vi "search_array_for_matches.vi"(9 "protocol selection ref":refnum<vi>, 10 "Protocol enum":T1, 11 "appended array":T2 {"Mode" items=["Modbus-1", "3"]}) -> (1 "Array of exists":bool[](array[boolean]), 2 "array of indexes":i32[](array[numeric]), 3 "exists?":bool, 4 "Switch Row":i32, 5 "Array of addresses":i32[](array[numeric]), 7 "all addresses":i32[](array[numeric]))   [LabVIEW 2016]
uses:
  Typedef/Array_of_Comm_mode_and_address_types.ctl
  Typedef/Comm_mode_and_address_type.ctl
  Typedef/Comm_mode_type_combo.ctl
  Typedef/Protocol_enum_type.ctl
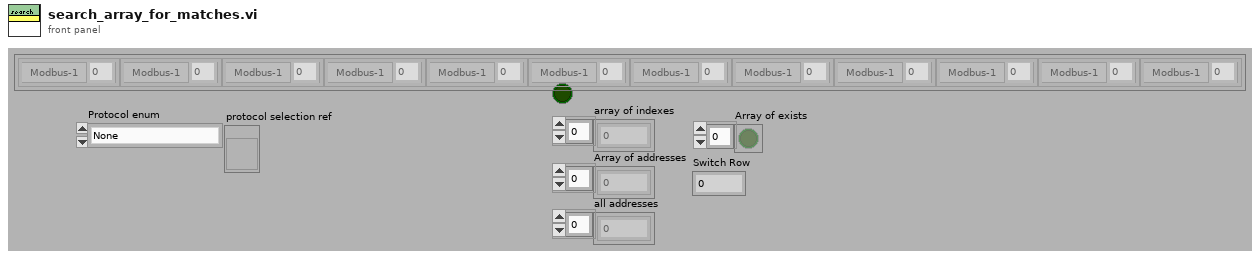
[diagram p1: front panel]
types:
  T1 = typedef "Protocol_enum_type.ctl" = enum16{"None", "MODBUS", "HART", "Fieldbus", "Profibus DP", "Profibus PA", "DeviceNET", "USB"}
  T2 = typedef "Array_of_Comm_mode_and_address_types.ctl" = T3[]
  T3 = typedef "Comm_mode_and_address_type.ctl" = cluster{"address":i32, "Mode":T4}
  T4 = typedef "Comm_mode_type_combo.ctl" = u16
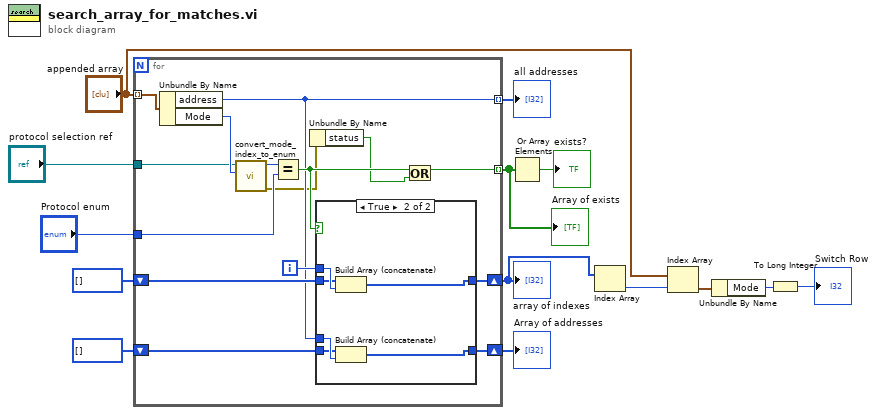
[diagram p0: block diagram]
diagram:
  n1 = for {
    tunnel: "appended array" -> [w29] mode=indexing
    tunnel: [w16] -> w14 mode=indexing
    tunnel: "Protocol enum" -> [w28]
    shift-right: [w25] -> w6
    shift-left: i32[] [] -> [w24]
    shift-right: [w23] -> w11
    shift-left: i32[] [] -> [w22]
    tunnel: [w21] -> w9 mode=indexing
    tunnel: "protocol selection ref" -> [w18]
    i -> [w26]
    n2 = Unbundle By Name(w29) -> ("address"=w21:i32, "Mode"=w20:T4)
    n3 = call "convert_mode_index_to_enum.vi"("index"=w20, "CtlRef"=w18) -> ("error out"=w17:errorcluster, "Protocol enum"=w19:T1)  [unwired: 6 in, 2 out]
    n4 = Equal?(x=w19, y=w28) -> (x = y?=w27:bool)
    n5 = Unbundle By Name(w17) -> ("status"=w15:bool)
    n6 = case shown="True" w27 {
      tunnel: w26 -> [_ w37]
      tunnel: [w31 w36] -> w25
      tunnel: w24 -> [w31 w35]
      tunnel: w21 -> [_ w34]
      tunnel: [w30 w33] -> w23
      tunnel: w22 -> [w30 w32]
      frame False {
      }
      frame True {
        n7 = Build Array (concatenate)(w35, w37) -> (w36:i32[])
        n8 = Build Array (concatenate)(w32, w34) -> (w33:i32[])
      }
    }
    n9 = Or(x=w27, y=w15) -> (x .or. y?=w16:bool)
  }
  "array of indexes" <- w6
  "Array of addresses" <- w11
  "all addresses" <- w9
  "Array of exists" <- w14
  n10 = Or Array Elements(Boolean array=w14) -> (logical OR=→"exists?":bool)
  n11 = Index Array(array=w6) -> (element=w4:i32)  [unwired: 1 in]
  n12 = Index Array(array="appended array", index=w4) -> (element=w3:T3)
  n13 = Unbundle By Name(w3) -> ("Mode"=w2:T4)
  n14 = To Long Integer(number=w2) -> (32bit integer=→"Switch Row":i32)
